vi "assemble.vi"(8 "error in (no error)":errorcluster, 11 "Table in":refnum<class "Table.lvclass">) -> (0 "error out":errorcluster, 2 "String":string="assembeld", 3 "Table out":refnum<class "Table.lvclass">)   [LabVIEW 2021, in "Table.lvclass"]
uses:
  Table.lvclass
  Table.lvclass/Table.ctl
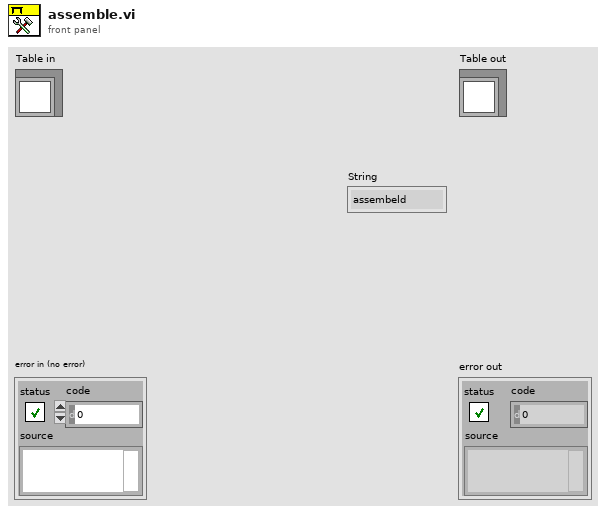
[diagram p1: front panel]
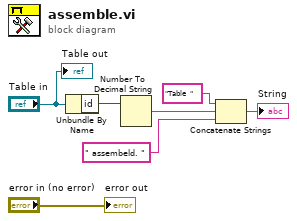
[diagram p0: block diagram]
diagram:
  n1 = Unbundle By Name("Table in") -> ("id"=w4:u32)
  n2 = Number To Decimal String(number=w4) -> (decimal integer string=w3:string)  [unwired: 1 in]
  n3 = Concatenate Strings("Table  ", w3, " assembeld. ") -> (→"String":string)
  "error out" <- "error in (no error)"
  "Table out" <- "Table in"
